vi "sub_calculate value.vi"(6 "Pixel/Line":u16(ring)=512 caption="X" items=["8"=8, "16"=16, "32"=32, "64"=64, "128"=128, "256"=256, "512"=512, "1024"=1024, "2048"=2048], 7 "Fill Fraction":dbl=0.85 min=0.1 max=0.97 step=0.01, 8 "Wave":enum16{"Triangle", "Sine", "Ramp"}(ring)=enum."Sine", 9 "X Frequency":dbl=3500.0, 11 "Acq. Sample Rate":dbl=120000000.0 caption="Sanple Rate Divider" format="%#_6p") -> (2 "Pixel Dwell":dbl=28000000.0 format="%#_3g", 3 "Point/Pixel":i32=28)   [LabVIEW 2015]
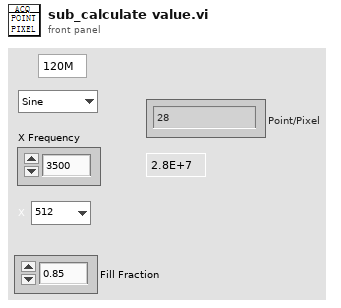
[diagram p1: front panel]
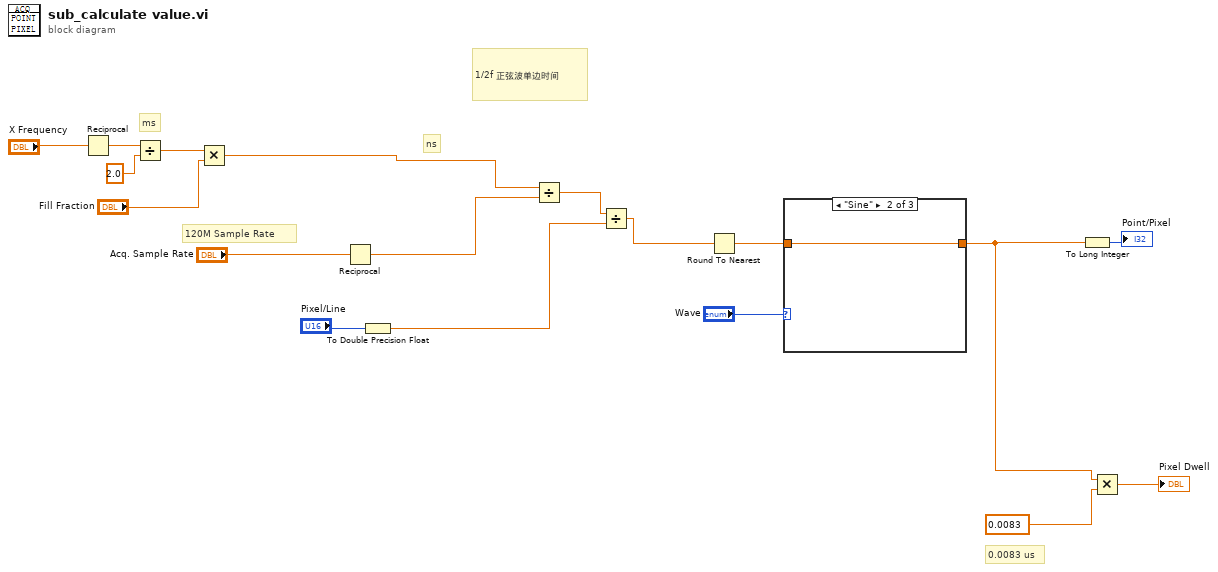
[diagram p0: block diagram]
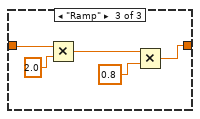
[diagram p3: hidden frame]
diagram:
  # "0.0083 us"
  # "120M Sample Rate"
  # "ns"
  # "ms"
  # "1/2f 正弦波单边时间"
  n1 = Reciprocal(x="X Frequency") -> (1/x=w11:dbl)
  n2 = Divide(x=w11, y=2.0) -> (x/y=w9:dbl)
  n3 = Multiply(x=w9, y="Fill Fraction") -> (x*y=w1:dbl)
  n4 = Reciprocal(x="Acq. Sample Rate") -> (1/x=w2:dbl)
  n5 = To Double Precision Float(number="Pixel/Line") -> (double precision float=w15:dbl)
  n6 = Divide(x=w1, y=w2) -> (x/y=w14:dbl)
  n7 = Divide(x=w14, y=w15) -> (x/y=w16:dbl)
  n8 = Round To Nearest(number=w16) -> (nearest integer value=w6:dbl)
  n9 = case shown="\"Sine\"" "Wave" {
    tunnel: [w19 w20 w25] -> w4
    tunnel: w6 -> [w19 w20 w24]
    frame "Triangle", Default {
    }
    frame "Sine" {
    }
    frame "Ramp" {
      n10 = Multiply(x=w24, y=2.0) -> (x*y=w21:dbl)
      n11 = Multiply(x=w21, y=0.8) -> (x*y=w25:dbl)
    }
  }
  n12 = To Long Integer(number=w4) -> (32bit integer=→"Point/Pixel":i32)
  n13 = Multiply(x=w4, y=0.0083) -> (x*y=→"Pixel Dwell":dbl)
